vi "Begin.vi"(8 "error in":errorcluster) -> (0 "error out":errorcluster)   [LabVIEW 2016]
doc: "Called before other user functions, this VI is expected to open initial I/O refnums, load in file data, and do all program initialization. Notice that the <B>error out</B> terminal is simply used for data flow. Wiring it to other structures or subVIs ensures that this VI runs first."
uses:
  Robot Global Data.vi
  <vilib>/Rock Robotics/WPI/DriverStation/WPI_DriverStationRobotMode2.ctl
  SwerveMotors.ctl
  <vilib>/Rock Robotics/WPI/ThirdParty/CanMotor/TalonSRX/WPI_CANTalonSRX_APIControlMode.ctl
  <vilib>/Rock Robotics/WPI/ThirdParty/CanMotor/TalonSRX/WPI_CANTalonSRX_APIFeedbackSelect.ctl
  DriveMotors.ctl
panel:
  in  "PID gains":T1={"proportional gain (Kc)"=5.0, "integral time (Ti, min)"=0.032, "derivative time (Td, min)"=0.0} {"derivative time (Td, min)" format="%.3f"; "integral time (Ti, min)" format="%.8f"; "proportional gain (Kc)" format="%.8f"}
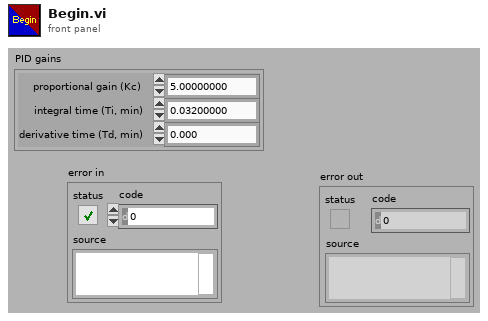
[diagram p1: front panel]
types:
  T1 = cluster{"proportional gain (Kc)":dbl, "integral time (Ti, min)":dbl, "derivative time (Td, min)":dbl}
  T2 = typedef "DriveMotors.ctl" = enum16{"Drive1", "Drive2", "Drive3", "Drive4"}
  T3 = typedef "WPI_DriverStationRobotMode2.ctl" = enum16{"Autonomous Disabled", "Autonomous Enabled", "Teleop Disabled", "Teleop Enabled", "Disconnected", "Finish", "Test Disabled", "Test Enabled", "Emergency Stopped"}
  T4 = typedef "WPI_CANTalonSRX_APIFeedbackSelect.ctl" = enum16{"Digital Quadrature Encoder", "Analog Potentiometer", "Analog Encoder", "Count on Quad-A (Rising-Edge)", "Count on Quad-A (Falling-Edge)", "CTR Magnetic Enc (Absolute)", "CTR Magnetic Enc (Relative)", "Pulse Width"}
  T5 = typedef "WPI_CANTalonSRX_APIControlMode.ctl" = enum8{"Percent VBus", "Speed", "Position", "Slave", "Unchanged / Invalid", "Voltage Compensation", "Current", "Motion Profile", "Motion Magic"}
  T6 = typedef "SwerveMotors.ctl" = enum16{"Swerve 1", "Swerve 2", "Swerve 3", "Swerve 4"}
  T7 = typedef "WPI_MotorControlDeviceRef.ctl" = cluster{"DeviceStatus":errorcluster, "Type":T8, "PWM":cluster{"PWM Channel":T9, "DeadBand":T10}, "CAN":cluster{"Device Number":u8, "SetOutput VI Ref":variant, "GetOutput VI Ref":variant, "Enable VI Ref":variant, "Disable VI Ref":variant, "Data":variant}, "Invert":bool}
  T8 = typedef "WPI_MotorControlType.ctl" = enum16{"PWM", "CAN"}
  T9 = typedef "FPGA_DIOPWMChannel.ctl" = enum8{"PWM 0", "PWM 1", "PWM 2", "PWM 3", "PWM 4", "PWM 5", "PWM 6", "PWM 7", "PWM 8", "PWM 9", "PWM MXP 0", "PWM MXP 1", "PWM MXP 2", "PWM MXP 3", "PWM MXP 4", "PWM MXP 5", "PWM MXP 6", "PWM MXP 7", "PWM MXP 8", "PWM MXP 9", "Invalid"}
  T10 = typedef "WPI_PWMDeadband.ctl" = cluster{"Name":string, "maxPositivePwm":i32, "minPositivePwm":i32, "centerPwm":i32, "maxNegativePwm":i32, "minNegativePwm":i32, "angularRange":u16}
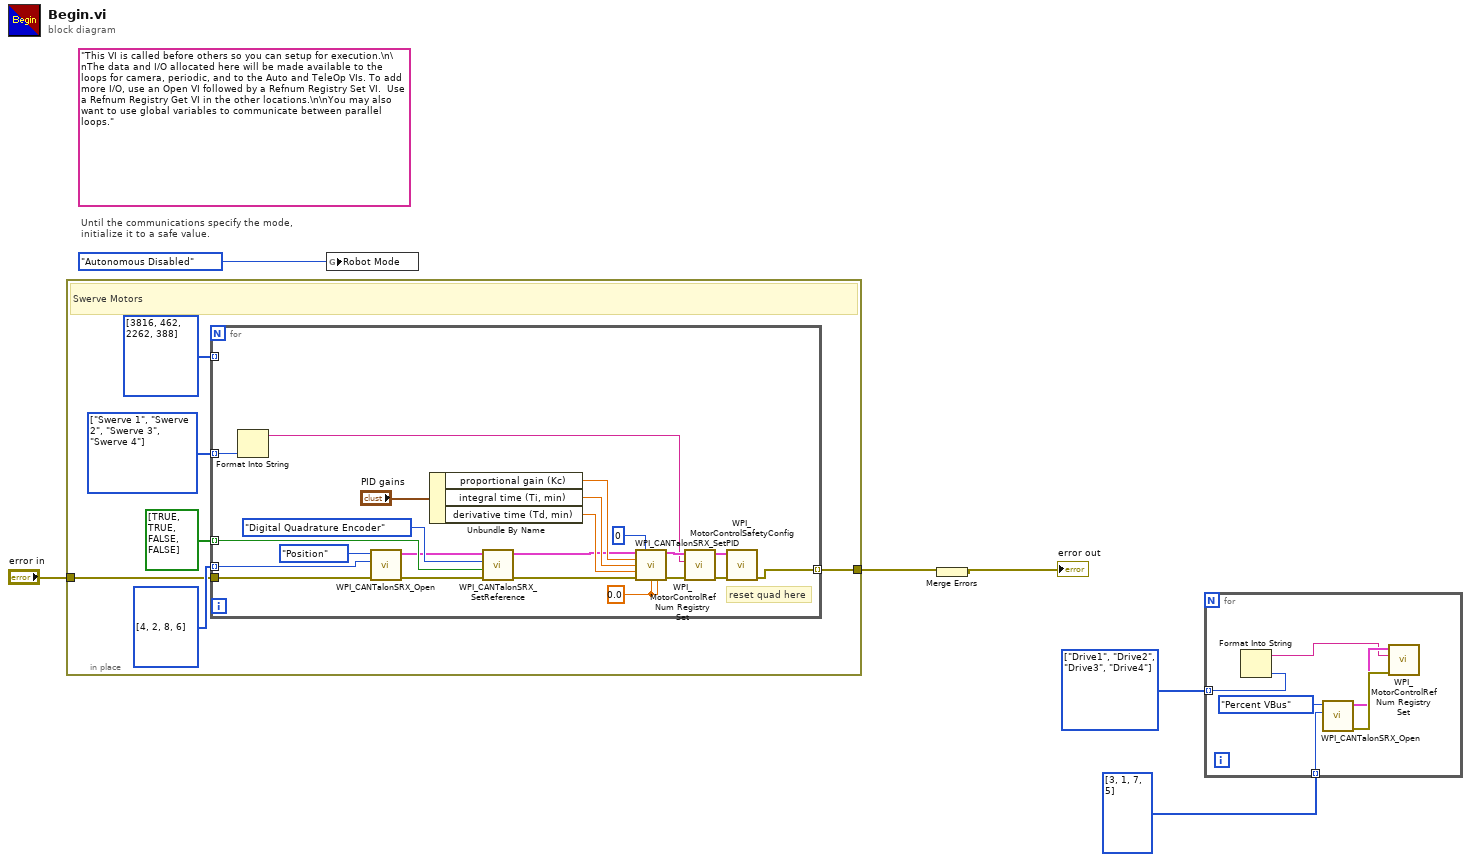
[diagram p0: block diagram]
diagram:
  w2 = T2[] [enum."Drive1", enum."Drive2", enum."Drive3", enum."Drive4"] items=["Drive1", "Drive2", "Drive3", "Drive4"]
  (unwired) "This VI is called before others so you can setup for execution.\n\nThe data and I/O allocated here will be made available to the loops for camera, periodic, and to the Auto and TeleOp VIs. To add more I/O, use an Open VI followed by a Refnum Registry Set VI.  Use a Refnum Registry Get VI in the other locations.\n\nYou may also want to use global variables to communicate between parallel loops."
  # "Until the communications specify the mode,\ninitialize it to a safe value."
  n1 = in-place {
    in-place-border: "error in" -> [w9]
    in-place-border: [w7] -> w4
    w12 = T6[] [enum."Swerve 1", enum."Swerve 2", enum."Swerve 3", enum."Swerve 4"] items=["Swerve 1", "Swerve 2", "Swerve 3", "Swerve 4"]
    # "Swerve Motors"
    n2 = for {
      tunnel: w12 -> [w25] mode=indexing
      tunnel: u8[] [4, 2, 8, 6] -> [w30] mode=indexing
      tunnel: w9 -> [w28]
      tunnel: bool[] [TRUE, TRUE, FALSE, FALSE] -> [w18] mode=indexing
      tunnel: i32[] [3816, 462, 2262, 388] -> [_] mode=indexing
      tunnel: [w13] -> w7 mode=indexing
      w19 = 0.0
      # "reset quad here"
      n3 = Format Into String(w25) -> (resulting string=w24:string)  [unwired: 3 in, 1 out]
      n4 = call <vilib>:"WPI_CANTalonSRX_Open.vi"("error in"=w28, "Device Number"=w30, "Control Mode"=WPI_CANTalonSRX_APIControlMode."Position") -> ("error out"=w33:errorcluster, "CAN Talon SRX Ref"=w16:T7)  [unwired: 7 in]
      n5 = Unbundle By Name("PID gains") -> ("proportional gain (Kc)"=w22:dbl, "integral time (Ti, min)"=w21:dbl, "derivative time (Td, min)"=w20:dbl)
      n6 = call <vilib>:"WPI_CANTalonSRX_SetReference.vi"("error in (no error)"=w33, "Reverse Feedback Sensor"=w18, "Feedback Reference"=WPI_CANTalonSRX_APIFeedbackSelect."Digital Quadrature Encoder", "CAN Talon SRX Ref"=w16) -> ("error out"=w32:errorcluster, "CAN Talon SRX Ref"=w15:T7)  [unwired: 6 in]
      n7 = call <vilib>:"WPI_CANTalonSRX_SetPID.vi"("CAN Talon SRX Ref"=w15, "Parameter Slot"=u8 0, "P"=w22, "I"=w21, "D"=w20, "error in (no error)"=w32, "I Zone"=w19, "Ramp Rate"=w19) -> ("CAN Talon SRX Ref"=w26:T7, "error out"=w31:errorcluster)  [unwired: 6 in]
      n8 = call <vilib>:"WPI_MotorControlRefNum Registry Set.vi"("error in (no error)"=w31, "refnum name"=w24, "MotorControlDevRef"=w26) -> ("error out"=w34:errorcluster, "MotorControlDevRef"=w27:T7)  [unwired: 7 in]
      n9 = call <vilib>:"WPI_MotorControlSafetyConfig.vi"("error in (no error)"=w34, "MotorControlDevRef"=w27) -> ("error out"=w13:errorcluster)  [unwired: 8 in, 1 out]
    }
  }
  n10 = global write "Robot Global Data.vi" "Robot Mode"(WPI_DriverStationRobotMode2."Autonomous Disabled" ("Robot Mode")) -> ()
  n11 = Merge Errors(w4) -> (→"error out":errorcluster)
  n12 = for {
    tunnel: w2 -> [w40] mode=indexing
    tunnel: i32[] [3, 1, 7, 5] -> [w39] mode=indexing
    n13 = Format Into String(w40) -> (resulting string=w36:string)  [unwired: 3 in, 1 out]
    n14 = call <vilib>:"WPI_CANTalonSRX_Open.vi"("Device Number"=w39, "Control Mode"=WPI_CANTalonSRX_APIControlMode."Percent VBus") -> ("error out"=w38:errorcluster, "CAN Talon SRX Ref"=w37:T7)  [unwired: 8 in]
    n15 = call <vilib>:"WPI_MotorControlRefNum Registry Set.vi"("error in (no error)"=w38, "refnum name"=w36, "MotorControlDevRef"=w37) -> ()  [unwired: 7 in, 2 out]
  }
